vi "WriteBacklogToFile.vi"(8 "error in (no error)":errorcluster, 10 "backlog messages":T1[](array[typedef]), 11 "log dir":path) -> (0 "error out":errorcluster)   [LabVIEW 2017, in "TracePointSynchronizer.lvlib"]
uses:
  <vilib>/addons/InsightCM/Devices/Shared/Common/TracePointSynchronizer/TracePointSynchronizer.lvlib
  <vilib>/addons/InsightCM/MessageBus/Base/controls/Message.ctl
  <vilib>/addons/InsightCM/MessageBus/Base/controls/MessageHeader.ctl
  <vilib>/addons/InsightCM/MessageBus/Base/controls/KeyValuePair.ctl
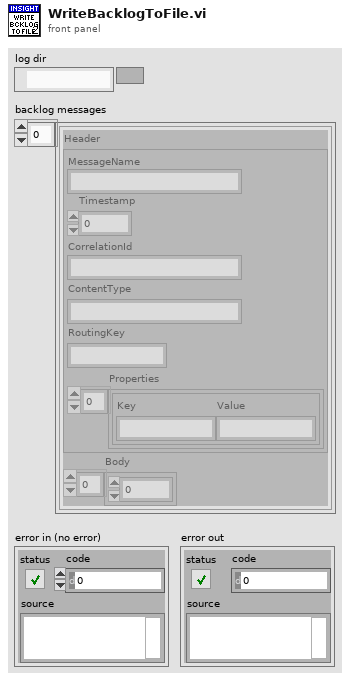
[diagram p1: front panel]
types:
  T1 = typedef "Message.ctl" = cluster{"Header":T2, "Body":u8[]}
  T2 = typedef "MessageHeader.ctl" = cluster{"MessageName":string, "Timestamp":i64, "CorrelationId":string, "ContentType":string, "RoutingKey":string, "Properties":T3[]}
  T3 = typedef "KeyValuePair.ctl" = cluster{"Key":string, "Value":string}
  T4 = enum16{"open", "replace", "create", "open or create", "replace or create", "replace or create with confirmation"}
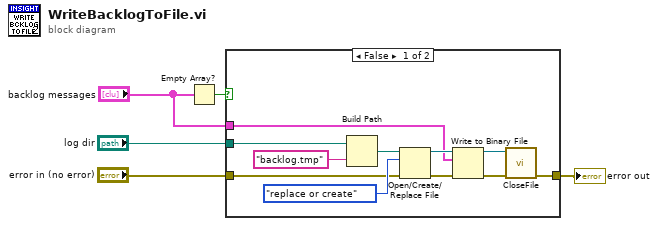
[diagram p0: block diagram]
diagram:
  n1 = Empty Array?(array="backlog messages") -> (empty?=w3:bool)
  n2 = case shown="False" w3 {
    tunnel: [w6 w17] -> w5
    tunnel: "error in (no error)" -> [w13 w17]
    tunnel: "log dir" -> [w10 _]
    tunnel: "backlog messages" -> [w9 _]
    frame False {
      n3 = Build Path(base path=w10, name or relative path="backlog.tmp") -> (appended path=w11:path)
      n4 = Open/Create/Replace File(file path (use dialog)=w11, error in=w13, operation (0:open)=T4."replace or create") -> (refnum out=w15:refnum<file>, error out=w14:errorcluster)  [unwired: 3 in, 1 out]
      n5 = Write to Binary File(file (use dialog)=w15, data=w9, error in=w14) -> (refnum out=w8:refnum<file>, error out=w7:errorcluster)  [unwired: 3 in, 1 out]
      n6 = call <vilib>:"CloseFile.vi"("error in (no error)"=w7, "file reference"=w8) -> ("error out"=w6:errorcluster)  [unwired: 9 in]
    }
    frame True {
    }
  }
  "error out" <- w5
